vi "MIF_auto_X_txt-de-obs.vi"(1 "xt-obs":string[](array[string])) -> (0 "xt-MIF":string[](array[string]))   [LabVIEW 2010, in "lv_02.lvlib"]
doc: "Pour une variable qualtitative (txt), à partir du tableau xt-obs des n observations, le VI retourne un tableau xt-MIF des valeurs distinctes observées"
uses:
  lv_02.lvlib
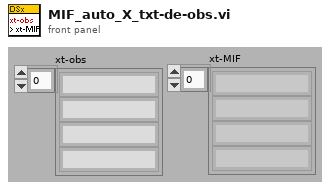
[diagram p1: front panel]
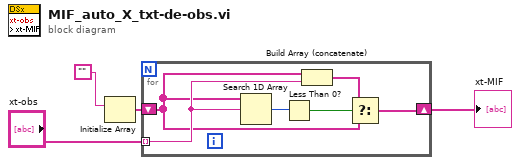
[diagram p0: block diagram]
diagram:
  n1 = Initialize Array("") -> (w2:string[])  [unwired: 1 in]
  n2 = for {
    tunnel: "xt-obs" -> [w9] mode=indexing
    shift-right: [w6] -> w4
    shift-left: w2 -> [w7]
    n3 = Search 1D Array(1D array=w7, element=w9) -> (index of element=w10:i32)  [unwired: 1 in]
    n4 = Less Than 0?(x=w10) -> (x < 0?=w5:bool)
    n5 = Build Array (concatenate)(w7, w9) -> (w8:string[])
    n6 = Select(t=w8, s=w5, f=w7) -> (s? t:f=w6:string[])
  }
  "xt-MIF" <- w4
